vi "Calculated result.vi"(9 "Operator Array":string[](array[string]), 11 "Number Array":dbl[](array[numeric])) -> (3 "Result":dbl format="%#.12g")   [LabVIEW 2019]
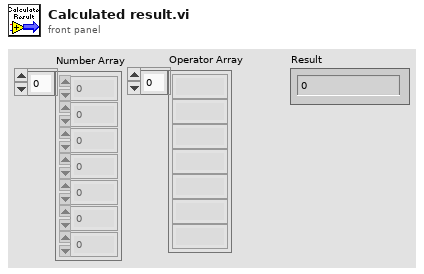
[diagram p1: front panel]
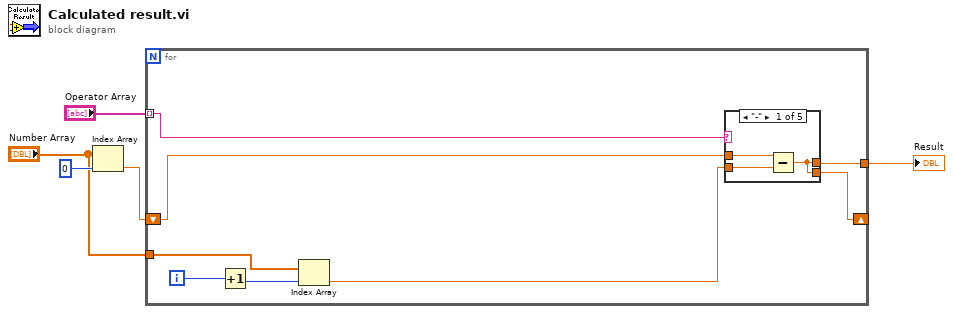
[diagram p0: block diagram]
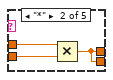
[diagram p2: hidden frame]
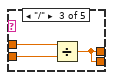
[diagram p3: hidden frame]
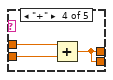
[diagram p4: hidden frame]
diagram:
  n1 = Index Array(array="Number Array", index=0) -> (element=w2:dbl)
  n2 = for {
    tunnel: "Operator Array" -> [w13] mode=indexing
    tunnel: [w12] -> w4
    shift-right: [w10] -> _
    shift-left: w2 -> [w11]
    tunnel: "Number Array" -> [w7]
    i -> [w9]
    n3 = Increment(x=w9) -> (x+1=w8:i32)
    n4 = Index Array(array=w7, index=w8) -> (element=w6:dbl)
    n5 = case shown="\"-\"" w13 {
      tunnel: [w16 w19 w22 w25 w26] -> w12
      tunnel: [w16 w19 w22 w25 w26] -> w10
      tunnel: w11 -> [w15 w18 w21 w24 w26]
      tunnel: w6 -> [w14 w17 w20 w23 _]
      frame "-" {
        n6 = Subtract(x=w15, y=w14) -> (x-y=w16:dbl)
      }
      frame "*" {
        n7 = Multiply(x=w18, y=w17) -> (x*y=w19:dbl)
      }
      frame "/" {
        n8 = Divide(x=w21, y=w20) -> (x/y=w22:dbl)
      }
      frame "+" {
        n9 = Add(x=w24, y=w23) -> (x+y=w25:dbl)
      }
      frame Default {
      }
    }
  }
  "Result" <- w4
